vi "CheckRunProbe.vi"(0 "UiDefinition":T1) -> ()   [LabVIEW 2020]
uses:
  UIReferences.ctl
  D:/LabviewDXFViewer/LabviewDXFViewer/bin/Release/LabviewDXFViewer.exe
  LabviewDXFViewer/bin/Release/LabviewDXFViewer.exe
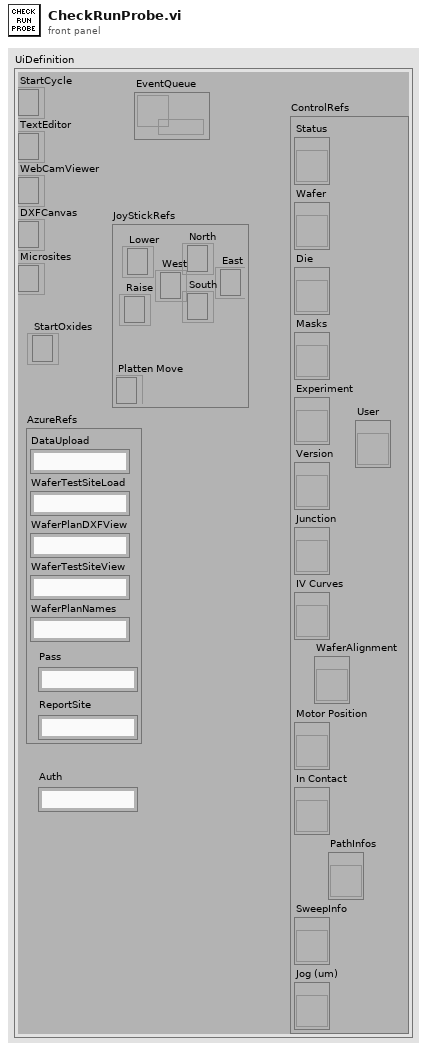
[diagram p1: front panel]
types:
  T1 = typedef "UIReferences.ctl" = cluster{"StartCycle":refnum<k24>, "TextEditor":refnum<k24>, "WebCamViewer":refnum<k24>, "DXFCanvas":refnum<k24>, "Microsites":refnum<k24>, "JoyStickRefs":cluster{"North":refnum<k24>, "Lower":refnum<k24>, "Raise":refnum<k24>, "Platten Move":refnum<k24>, "West":refnum<k24>, "East":refnum<k24>, "South":refnum<k24>}, "AzureRefs":cluster{"DataUpload":string, "WaferTestSiteLoad":string, "WaferPlanDXFView":string, "WaferTestSiteView":string, "WaferPlanNames":string, "Pass":string, "ReportSite":string}, "ControlRefs":cluster{"Status":refnum<vi>, "Wafer":refnum<vi>, "Die":refnum<vi>, "Masks":refnum<vi>, "Experiment":refnum<vi>, "Version":refnum<vi>, "Junction":refnum<vi>, "IV Curves":refnum<vi>, "Motor Position":refnum<vi>, "In Contact":refnum<vi>, "SweepInfo":refnum<vi>, "Jog (um)":refnum<vi>, "PathInfos":refnum<vi>, "User":refnum<vi>, "WaferAlignment":refnum<vi>}, "EventQueue":refnum<queue>, "StartOxides":refnum<k24>, "Auth":string}
  T2 = cluster{"Status":refnum<vi>, "Wafer":refnum<vi>, "Die":refnum<vi>, "Masks":refnum<vi>, "Experiment":refnum<vi>, "Version":refnum<vi>, "Junction":refnum<vi>, "IV Curves":refnum<vi>, "Motor Position":refnum<vi>, "In Contact":refnum<vi>, "SweepInfo":refnum<vi>, "Jog (um)":refnum<vi>, "PathInfos":refnum<vi>, "User":refnum<vi>, "WaferAlignment":refnum<vi>}
  T3 = typedef "WaferAlignmentType.ctl" = cluster{"Wafer Units to microns":dbl, "Rotation Misalign":dbl[], "Scale Misalign":dbl, "Steps Per micron":dbl, "Position 1":i32[], "Position 2":i32[], "Lift Distance":i32, "Position 3":i32[], "Jog Height":i32}
  T4 = cluster{"Die":string, "Wafer":string, "Path":path, "url":string, "Experiment":string, "Version":string, "user":string}
  T5 = cluster{"Current Range":dbl, "Source Measure Unit Channel (0: Channel A)":i32, "Waveform":waveform(dbl), "VISA resource name":refnum<visa-resource-name>, "CodeText":string}
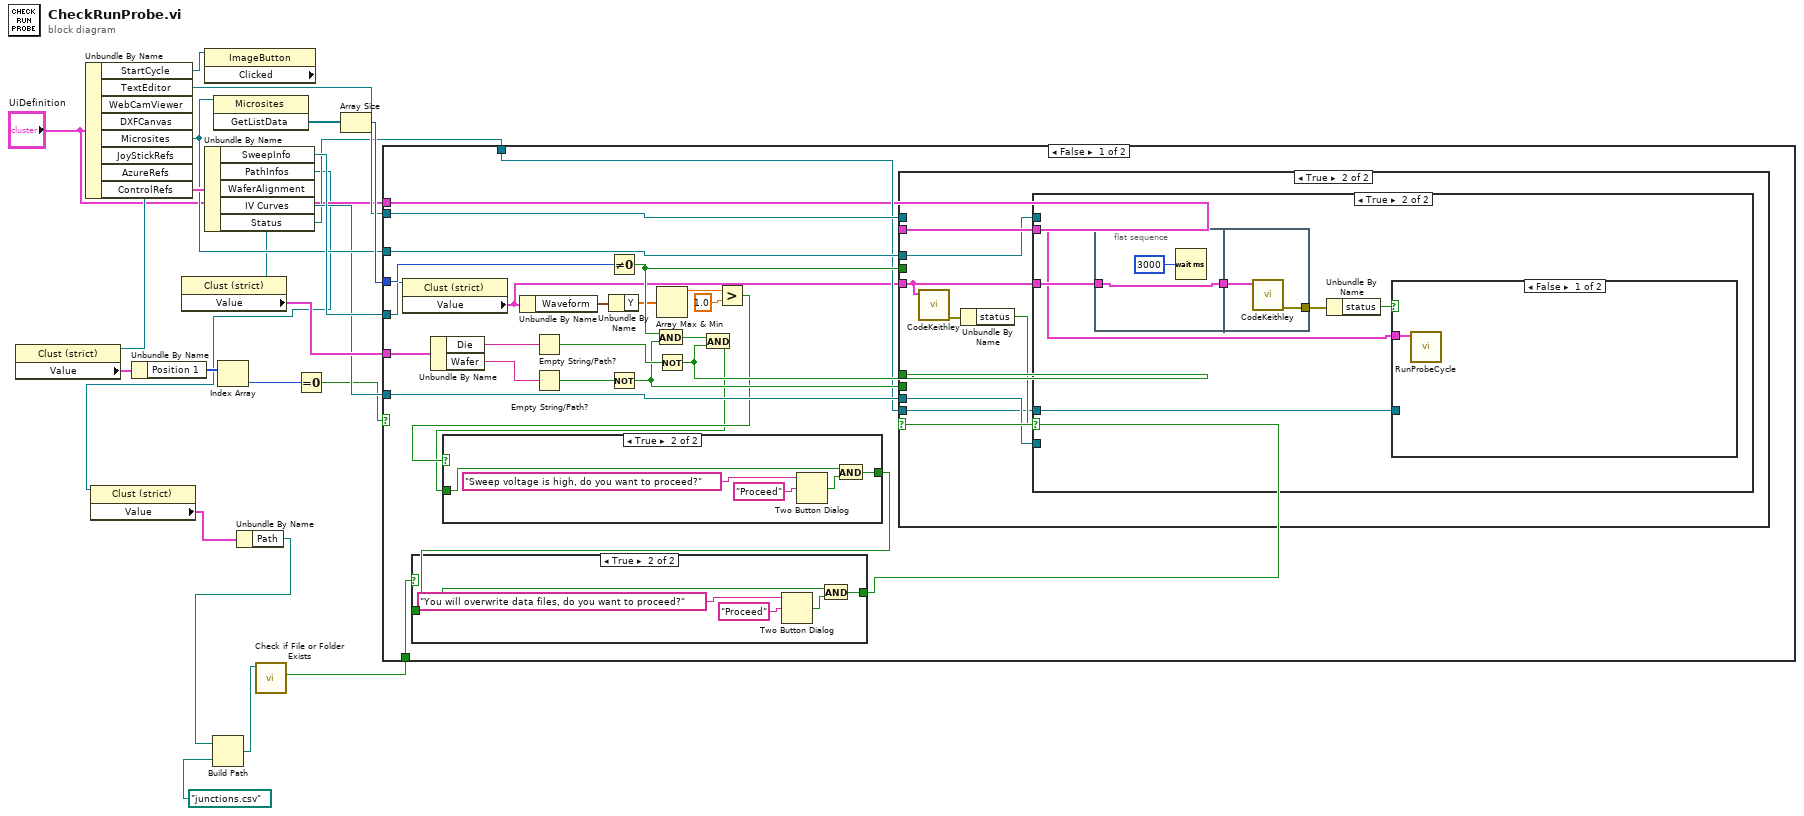
[diagram p0: block diagram]
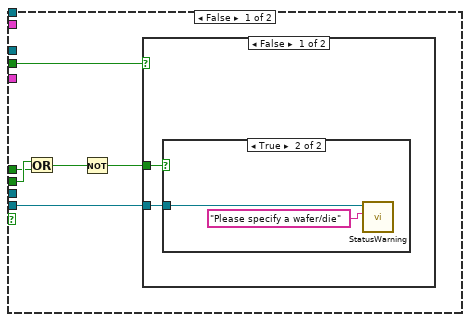
[diagram p4: hidden frame]
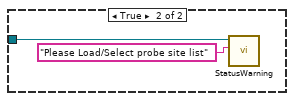
[diagram p6: hidden frame]
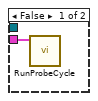
[diagram p7: hidden frame]
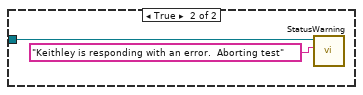
[diagram p8: hidden frame]
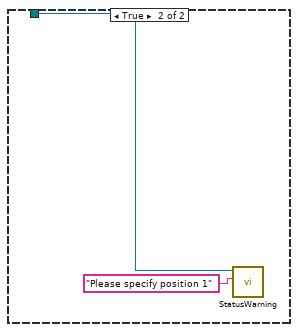
[diagram p9: hidden frame]
diagram:
  n1 = Unbundle By Name("UiDefinition") -> ("StartCycle"=w10:refnum<k24>, "TextEditor"=w14:refnum<k24>, "Microsites"=w15:refnum<k24>, "ControlRefs"=w20:T2)  [unwired: 4 out]
  n2 = property class="ImageButton" props=["Clicked"](reference=w10) -> ()  [unwired: 1 in, 3 out]
  n3 = Unbundle By Name(w20) -> ("SweepInfo"=w19:refnum<vi>, "PathInfos"=w6:refnum<vi>, "WaferAlignment"=w17:refnum<vi>, "IV Curves"=w13:refnum<vi>, "Status"=w12:refnum<vi>)
  n4 = property class="Clust (strict)"(reference=w17) -> ("Value"=w16:T3)  [unwired: 1 in, 2 out]
  n5 = property class="Clust (strict)"(reference=w6) -> ("Value"=w5:T4)  [unwired: 1 in, 2 out]
  n6 = Unbundle By Name(w16) -> ("Position 1"=w9:i32[])
  n7 = property class="Clust (strict)"(reference=w6) -> ("Value"=w18:T4)  [unwired: 1 in, 2 out]
  n8 = invoke class="Microsites" method="GetListData"(reference=w15) -> ("GetListData"=w21:refnum<k24>[])  [unwired: 2 in, 2 out]
  n9 = Index Array(array=w9) -> (element=w8:i32)  [unwired: 1 in]
  n10 = Unbundle By Name(w5) -> ("Path"=w2:path)
  n11 = Build Path(base path=w2, name or relative path=path "junctions.csv") -> (appended path=w3:path)
  n12 = call <vilib>:"Check if File or Folder Exists.vi"("path"=w3) -> ("file or folder exists?"=w1:bool)  [unwired: 8 in, 2 out]
  n13 = Equal To 0?(x=w8) -> (x = 0?=w7:bool)
  n14 = Array Size(array=w21) -> (size(s)=w22:i32)
  n15 = case shown="False" w7 {
    tunnel: w22 -> [w48 _]
    tunnel: w19 -> [w39 _]
    tunnel: w18 -> [w38 _]
    tunnel: w15 -> [w37 _]
    tunnel: w14 -> [w36 _]
    tunnel: w13 -> [w35 _]
    tunnel: w12 -> [w34 w94]
    tunnel: "UiDefinition" -> [w33 _]
    tunnel: w1 -> [w23 _]
    frame False {
      n16 = property class="Clust (strict)"(reference=w39) -> ("Value"=w26:T5)  [unwired: 1 in, 2 out]
      n17 = Unbundle By Name(w38) -> ("Die"=w40:string, "Wafer"=w41:string)
      n18 = Unbundle By Name(w26) -> ("Waveform"=w32:waveform(dbl))
      n19 = Empty String/Path?(string/path=w40) -> (empty?=w44:bool)
      n20 = Empty String/Path?(string/path=w41) -> (empty?=w45:bool)
      n21 = Not Equal To 0?(x=w48) -> (x != 0?=w46:bool)
      n22 = Unbundle By Name(w32) -> ("Y"=w31:dbl[])
      n23 = Not(x=w45) -> (.not. x?=w42:bool)
      n24 = And(x=w46, y=w42) -> (x .and. y?=w47:bool)
      n25 = Array Max & Min(array=w31) -> (max value=w30:dbl)  [unwired: 3 out]
      n26 = Not(x=w44) -> (.not. x?=w43:bool)
      n27 = And(x=w47, y=w43) -> (x .and. y?=w27:bool)
      n28 = Greater?(x=w30, y=1.0) -> (0:w28:bool)
      n29 = case shown="True" w28 {
        tunnel: w27 -> [w55 w56]
        tunnel: [w55 w57] -> w25
        frame False {
        }
        frame True {
          n30 = Two Button Dialog(message="Sweep voltage is high, do you want to proceed?", 2:"Proceed" ("T button name (\"OK\")")) -> (T button?=w58:bool)  [unwired: 1 in]
          n31 = And(x=w56, y=w58) -> (x .and. y?=w57:bool)
        }
      }
      n32 = case shown="True" w23 {
        tunnel: w25 -> [w49 w50]
        tunnel: [w49 w51] -> w24
        frame False {
        }
        frame True {
          n33 = Two Button Dialog(message="You will overwrite data files, do you want to proceed?", 2:"Proceed" ("T button name (\"OK\")")) -> (T button?=w52:bool)  [unwired: 1 in]
          n34 = And(x=w50, y=w52) -> (x .and. y?=w51:bool)
        }
      }
      n35 = case shown="True" w24 {
        tunnel: w46 -> [w66 _]
        tunnel: w42 -> [w65 _]
        tunnel: w43 -> [w64 _]
        tunnel: w36 -> [_ _]
        tunnel: w37 -> [_ w79]
        tunnel: w26 -> [_ w73]
        tunnel: w35 -> [_ w78]
        tunnel: w34 -> [w61 w75]
        tunnel: w33 -> [_ w74]
        frame False {
          n36 = Or(x=w65, y=w64) -> (x .or. y?=w63:bool)
          n37 = Not(x=w63) -> (.not. x?=w62:bool)
          n38 = case shown="False" w66 {
            tunnel: w62 -> [w68 _]
            tunnel: w61 -> [w67 w71]
            frame False {
              n39 = case shown="True" w68 {
                tunnel: w67 -> [_ w69]
                frame False {
                }
                frame True {
                  n40 = call "StatusWarning.vi"("Text.Text"="Please specify a wafer/die", "String in"=w69) -> ()  [unwired: 10 in]
                }
              }
            }
            frame True {
              n41 = call "StatusWarning.vi"("Text.Text"="Please Load/Select probe site list", "String in"=w71) -> ()  [unwired: 10 in]
            }
          }
        }
        frame True {
          n42 = call "CodeKeithley.vi"("SweepInfo"=w73) -> ("error out"=w77:errorcluster)  [unwired: 10 in]
          n43 = Unbundle By Name(w77) -> ("status"=w76:bool)
          n44 = case shown="True" w76 {
            tunnel: w79 -> [_ _]
            tunnel: w78 -> [_ _]
            tunnel: w75 -> [_ w86]
            tunnel: w74 -> [w80 w82]
            tunnel: w73 -> [_ w85]
            frame False {
              n45 = call "RunProbeCycle.vi"("UiDefinition"=w80) -> ()  [unwired: 10 in]
            }
            frame True {
              n46 = flat-sequence {
                tunnel: w85 -> [w88]
                tunnel: [w88] -> w81
                tunnel: [w89] -> w84
                tunnel: w81 -> [w90]
                frame #0 {
                  n47 = Wait (ms)(milliseconds to wait=u32 3000) -> ()  [unwired: 1 out]
                }
                frame #1 {
                  n48 = call "CodeKeithley.vi"("SweepInfo"=w90) -> ("error out"=w89:errorcluster)  [unwired: 10 in]
                }
              }
              n49 = Unbundle By Name(w84) -> ("status"=w83:bool)
              n50 = case shown="False" w83 {
                tunnel: w86 -> [_ w92]
                tunnel: w82 -> [w91 _]
                frame False {
                  n51 = call "RunProbeCycle.vi"("UiDefinition"=w91) -> ()  [unwired: 10 in]
                }
                frame True {
                  n52 = call "StatusWarning.vi"("Text.Text"="Keithley is responding with an error.  Aborting test", "String in"=w92) -> ()  [unwired: 10 in]
                }
              }
            }
          }
        }
      }
    }
    frame True {
      n53 = call "StatusWarning.vi"("Text.Text"="Please specify position 1", "String in"=w94) -> ()  [unwired: 10 in]
    }
  }
